vi "PTScanner.form scan.vi"(0 "i ref in":refnum<vi>, 5 "error in (no error)":errorcluster) -> (14 "i ref out":refnum<vi>, 19 "error out":errorcluster)   [LabVIEW 2014, in "PTScanner.lvlib"]
uses:
  PTScanner.lvlib
  CSlibraries-extern/DimLVEvent/LVDimInterface/LVDimInterface.lvlib
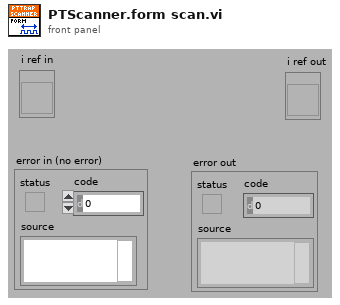
[diagram p1: front panel]
types:
  T1 = typedef "PTScanner.lvlib/PTScanner.i attribute.ctl" = cluster{"Object cmds":T2[], "Steps":cluster{"Finished":bool, "cmd setup":T3[]}[], "curStep":i32, "DIM IDs":cluster{"AllFinished":i32, "Finished":i32, "curStep":i32, "nofSteps":i32, "NomValues":i32[], "1D-Min":i32, "1D-Max":i32, "Dimensions":i32, "MaxDimensions":i32, "ScanedDeviceNames":i32[]}, "All Finished":bool, "DIMs in use":string[], "Running":bool, "Scan Delay":u32, "loop":bool, "Paused":bool, "Formed":bool}
  T2 = typedef "PTScanner.lvlib/PTScanner.obj parameters.ctl" = cluster{"object":string, "DIM address":string, "method":string, "data descriptor":string, "method parameters":cluster{"Name":string, "Descr":string, "Value":string, "Value?":bool}[], "Call Mode":enum16{"Simple DIM", "Synchronous"}, "actValue":dbl, "Centroid":dbl, "Minus Delta":dbl, "Plus Delta":dbl, "increment":dbl, "DIM Status":cluster{"no link":bool, "quality":i32, "Time Stamp":timestamp}, "range":dbl, "DIMChannelIndex":i32}
  T3 = typedef "PTScanner.lvlib/PTScanner.step obj parameters.ctl" = cluster{"obj index":i32, "nomValue":dbl, "fulfilled":bool}
  T4 = cluster{"Finished":bool, "object's setup":T3[]}[]
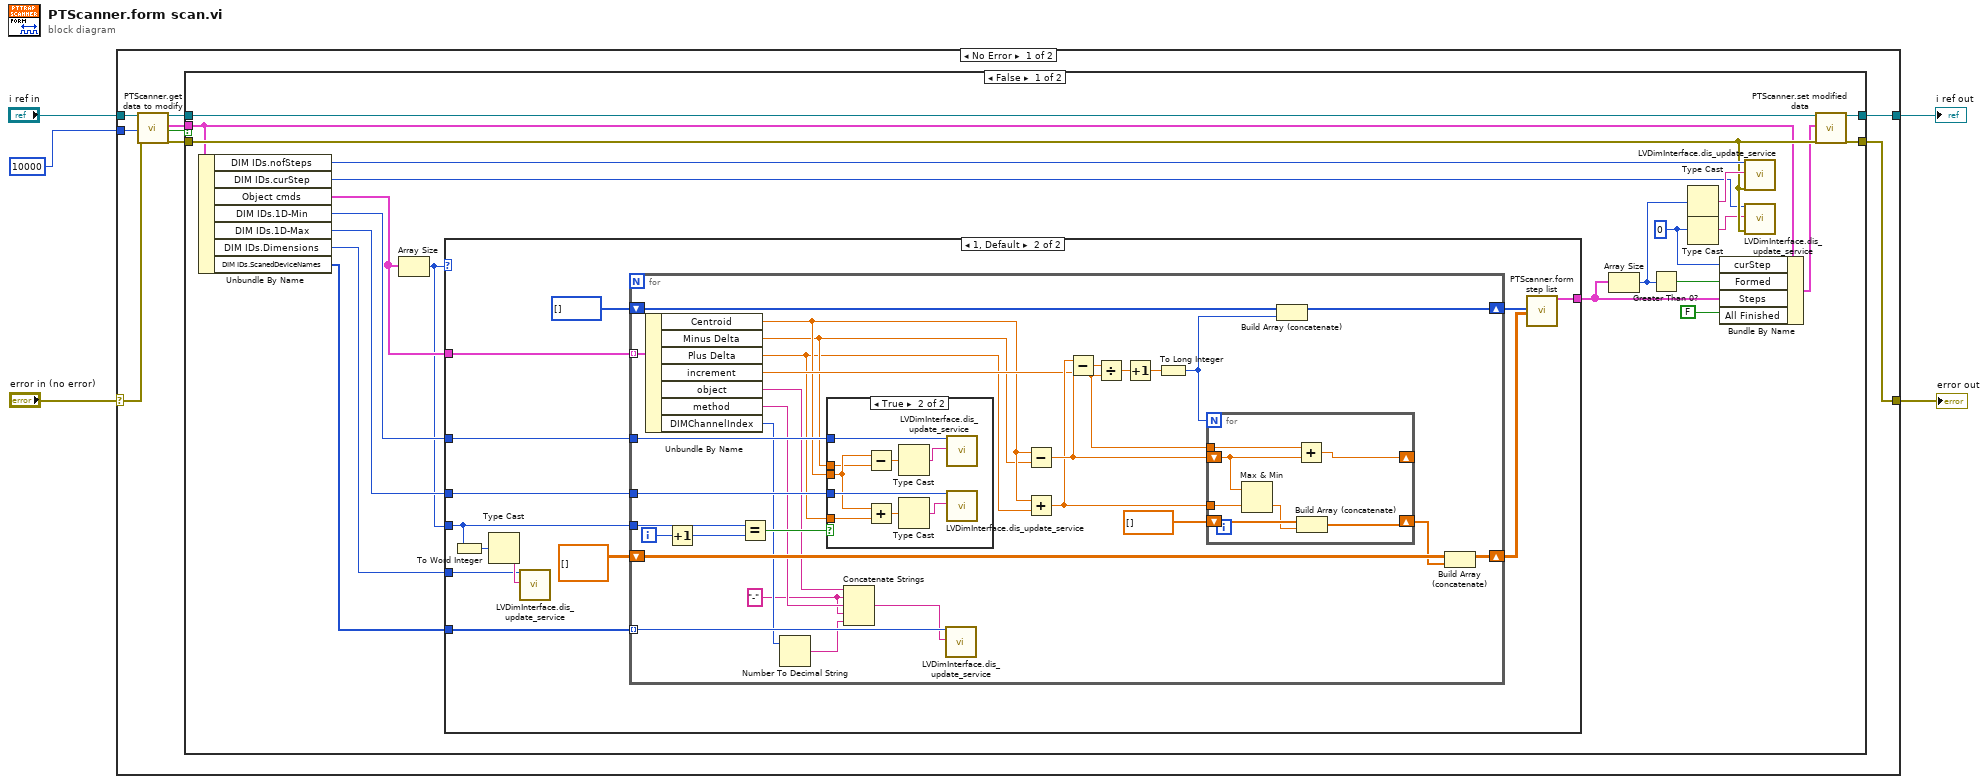
[diagram p0: block diagram]
diagram:
  n1 = case shown="No Error" "error in (no error)" {
    selector: "error in (no error)" -> [w13 w97]
    tunnel: [w10 w98] -> w4
    tunnel: "i ref in" -> [w14 w98]
    tunnel: [w7 w97] -> w2
    tunnel: 10000 -> [w12 _]
    frame No Error {
      n2 = call "PTScanner.get data to modify.vi"("i ref in"=w14, "ms timeout (10000)"=w12, "error in (no error)"=w13) -> ("i ref out"=w9:refnum<vi>, "i attribute"=w6:T1, "timed out"=w11:bool, "error out"=w8:errorcluster)  [unwired: 13 in]
      n3 = case shown="False" w11 {
        tunnel: [w35 w96] -> w10
        tunnel: w9 -> [w33 w96]
        tunnel: w8 -> [w25 w95]
        tunnel: [w34 w95] -> w7
        tunnel: w6 -> [w21 _]
        frame False {
          w22 = 0
          n4 = Unbundle By Name(w21) -> ("DIM IDs.nofSteps"=w29:i32, "DIM IDs.curStep"=w23:i32, "Object cmds"=w32:T2[], "DIM IDs.1D-Min"=w19:i32, "DIM IDs.1D-Max"=w18:i32, "DIM IDs.Dimensions"=w16:i32, "DIM IDs.ScanedDeviceNames"=w15:i32[])
          n5 = Array Size(array=w32) -> (size(s)=w17:i32)
          n6 = case shown="1, Default" w17 {
            tunnel: w32 -> [_ w44]
            tunnel: [_ w43] -> w30
            tunnel: w19 -> [_ w42]
            tunnel: w18 -> [_ w41]
            tunnel: w17 -> [_ w37]
            tunnel: w16 -> [_ w39]
            tunnel: w15 -> [_ w36]
            frame 0 {
            }
            frame 1, Default {
              n7 = To Word Integer(number=w37) -> (16bit integer=w38:i16)
              n8 = Type Cast(x=w38) -> (*(type *) &x=w40:string)  [unwired: 1 in]
              n9 = call "LVDimInterface.dis_update_service.vi"("my_serviceID"=w39, "data"=w40) -> ()  [unwired: 15 in, 3 out]
              n10 = for {
                tunnel: w44 -> [w78] mode=indexing
                shift-right: [w76] -> w45
                shift-left: dbl[][] [] ("Objects") -> [w77]
                shift-right: [w73] -> w46
                shift-left: i32[] [] ("Sizes") -> [w72]
                tunnel: w42 -> [w64]
                tunnel: w41 -> [w63]
                tunnel: w37 -> [w59]
                tunnel: w36 -> [w55] mode=indexing
                i -> [w58]
                w49 = "-" ("string")
                n11 = Unbundle By Name(w78) -> ("Centroid"=w62:dbl, "Minus Delta"=w61:dbl, "Plus Delta"=w60:dbl, "increment"=w66:dbl, "object"=w54:string, "method"=w53:string, "DIMChannelIndex"=w51:i32)
                n12 = Increment(x=w58) -> (x+1=w56:i32)
                n13 = Equal?(x=w59, y=w56) -> (x = y?=w57:bool)
                n14 = Number To Decimal String(number=w51) -> (decimal integer string=w50:string)  [unwired: 1 in]
                n15 = case shown="True" w57 {
                  tunnel: w64 -> [_ w87]
                  tunnel: w63 -> [_ w86]
                  tunnel: w62 -> [_ w81]
                  tunnel: w61 -> [_ w80]
                  tunnel: w60 -> [_ w79]
                  frame False {
                  }
                  frame True {
                    n16 = Subtract(x=w81, y=w80) -> (x-y=w82:dbl)
                    n17 = Add(x=w81, y=w79) -> (x+y=w83:dbl)
                    n18 = Type Cast(x=w82) -> (*(type *) &x=w85:string)  [unwired: 1 in]
                    n19 = Type Cast(x=w83) -> (*(type *) &x=w84:string)  [unwired: 1 in]
                    n20 = call "LVDimInterface.dis_update_service.vi"("my_serviceID"=w87, "data"=w85) -> ()  [unwired: 15 in, 3 out]
                    n21 = call "LVDimInterface.dis_update_service.vi"("my_serviceID"=w86, "data"=w84) -> ()  [unwired: 15 in, 3 out]
                  }
                }
                n22 = Concatenate Strings(w54, w49, w53, w49, w50) -> (w52:string)
                n23 = call "LVDimInterface.dis_update_service.vi"("my_serviceID"=w55, "data"=w52) -> ()  [unwired: 15 in, 3 out]
                n24 = Subtract(x=w62, y=w61) -> (x-y=w68:dbl)
                n25 = Add(x=w62, y=w60) -> (x+y=w67:dbl)
                n26 = Subtract(x=w67, y=w68) -> (x-y=w71:dbl)
                n27 = Divide(x=w71, y=w66) -> (x/y=w65:dbl)
                n28 = Increment(x=w65) -> (x+1=w70:dbl)
                n29 = To Long Integer(number=w70) -> (32bit integer=w69:i32)
                n30 = for {
                  N: w69 -> [_]
                  shift-right: [w93] -> w75
                  shift-left: dbl[] [] -> [w94]
                  shift-right: [w92] -> _
                  shift-left: w68 -> [w89]
                  tunnel: w67 -> [w91]
                  tunnel: w66 -> [w88]
                  n31 = Max & Min(x=w89, y=w91) -> (min(x,y)=w90:dbl)  [unwired: 1 out]
                  n32 = Add(x=w88, y=w89) -> (x+y=w92:dbl)
                  n33 = Build Array (concatenate)(w94, w90) -> (w93:dbl[])
                }
                n34 = Build Array (concatenate)(w72, w69) -> (w73:i32[])
                n35 = Build Array (concatenate)(w77, w75) -> (w76:dbl[][])
              }
              n36 = call "PTScanner.form step list.vi"("Sizes"=w46, "Object table"=w45) -> ("Steps out"=w43:T4)  [unwired: 17 in]
            }
          }
          n37 = Array Size(array=w30) -> (size(s)=w27:i32)
          n38 = Greater Than 0?(x=w27) -> (x > 0?=w28:bool)
          n39 = Type Cast(x=w27) -> (*(type *) &x=w26:string)  [unwired: 1 in]
          n40 = Type Cast(x=w22) -> (*(type *) &x=w24:string)  [unwired: 1 in]
          n41 = Bundle By Name(cluster=w21, "curStep"=w22, "Formed"=w28, "Steps"=w30, "All Finished"=FALSE) -> (w20:T1)
          n42 = call "LVDimInterface.dis_update_service.vi"("my_serviceID"=w29, "data"=w26, "error in (no error)"=w25) -> ()  [unwired: 14 in, 3 out]
          n43 = call "LVDimInterface.dis_update_service.vi"("my_serviceID"=w23, "data"=w24, "error in (no error)"=w25) -> ()  [unwired: 14 in, 3 out]
          n44 = call "PTScanner.set modified data.vi"("i ref in"=w33, "CLASS.i attribute"=w20, "error in (no error)"=w25) -> ("i ref out"=w35:refnum<vi>, "error out"=w34:errorcluster)  [unwired: 15 in]
        }
        frame True {
        }
      }
    }
    frame Error {
    }
  }
  "i ref out" <- w4
  "error out" <- w2
